vi "Pre Launch Init.vi"(11 "Actor wLauncher in":refnum<class "Actor wLauncher.lvclass">) -> (0 "error out":errorcluster, 3 "Actor wLauncher out":refnum<class "Actor wLauncher.lvclass">)   [LabVIEW 2017, in "Framework.lvlib" / "Actor wLauncher.lvclass"]
doc: "(<B>Filename</B>: Actor Framework.lvlib:Actor.lvclass:Pre Launch Init.vi)\n\nDefines behavior that occurs after the Launch Nested Actor method is invoked but before the actor's Actor Core method begins running.\n\nBy default, this method does nothing. A descendant class may override it to define behavior."
uses:
  Actor wLauncher.lvclass
  Actor wUI/Actor wUI.lvclass
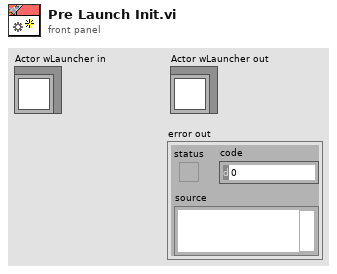
[diagram p1: front panel]
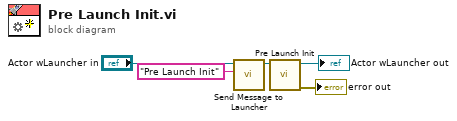
[diagram p0: block diagram]
diagram:
  n1 = call "Send Message to Launcher.vi"("Msg to Launcher"="Pre Launch Init", "Actor wLauncher in"="Actor wLauncher in") -> ("Actor wLauncher out"=w2:refnum<class "Actor wLauncher.lvclass">)  [unwired: 8 in, 1 out]
  n2 = call-parent "Pre Launch Init.vi"("Actor in"=w2) -> ("error out"=→"error out":errorcluster, "Actor out"=→"Actor wLauncher out":refnum<class "Actor wLauncher.lvclass">)  [unwired: 9 in]
